vi "Conversion Lookup Table.vi"(6 "command":enum16{"Set All", "Lookup Parameters"}(ring), 8 "error in (no error)":errorcluster {"code" min=0 max=0}, 9 "ID":u32, 10 "J1939 Process Parameters":T3={"J1939 XNET Settings"={"XNET Database"="", "XNET Cluster"="", "CAN Port"="", "Baud rate [Bd]"=0, "Termination"=0, "Incoming Rate"=0, "Outcoming Rate"=1, "Write Decimation"=1}, "Incoming Single Point Configuraiton"={"Incoming Single Point Frame"={"ID"=[], "Conversion"=[], "Channel Array Positions"=[], "Frame Length"=[]}, "Channel Pairs"={"Chan Refs"=[], "Previous Chan Values"=[]}, "Read FIFO"=refnum}, "Outgoing Cyclic Configuraiton"={"Outgoing Cyclic Frame"={"ID"=[], "Conversion"=[], "Channel Array Positions"=[], "Frame Length"=[], "Transmit Propreties"=[]}, "Channel Pairs"={"Block Data Refs"=[], "Previous Chan Values"=[]}, "Write FIFO"=refnum}, "J1939 Monitor Settings"={"J1939 Network Address"=0, "Name"=0}, "Simulated Addresses"=[], "Simulated Addresses LUT"=variant, "Name"=""} {"Simulated Addresses"."Simulated Addresses"."J1939 XNET Settings"."Name" format="%.0x"; "Simulated Addresses"."Simulated Addresses"."DM1 Data"."Data Reference" format="%.0x"; "Simulated Addresses"."Simulated Addresses"."DM1 Enable?"."Data Reference" format="%.0x"; "Simulated Addresses"."Simulated Addresses"."DM2 Data"."Data Reference" format="%.0x"; "Simulated Addresses"."Simulated Addresses"."DM2 Enable?"."Data Reference" format="%.0x"; "J1939 Monitor Settings"."Name" format="%.0x"; "Outgoing Cyclic Configuraiton"."Channel Pairs"."Block Data Refs"."Data Reference" format="%.0x"; "Outgoing Cyclic Configuraiton"."Outgoing Cyclic Frame"."Transmit Propreties"."Transmit Time" format="%#_p"; "J1939 XNET Settings"."Termination" items=["Off", "On"]; "Incoming Single Point Configuraiton"."Channel Pairs"."Chan Refs" format="%.0x"}, 11 "Scale Ref":T1) -> (0 "error out":errorcluster {"code" min=0 max=0}, 1 "Found?":bool, 2 "Parameters":T2, 3 "Scale Ref out":T1)   [LabVIEW 2015, in "J1939 Addon Engine.lvlib"]
uses:
  J1939 Addon Engine.lvlib
  Types/Process Parameters.ctl
  Shared/Types/XNET Settings.ctl
  Types/Incoming Single Point Configuration.ctl
  Types/Incoming Single Point Frame Pairs.ctl
  Shared/Types/Incoming Single Point Channel Pairs.ctl
  <vilib>/NI Veristand/Custom Device API/Data Reference.ctl
  Types/Outgoing Cyclic Configuration.ctl
  Types/Outgoing Cyclic Frame Pairs.ctl
  Shared/Types/XNET Frame Event Properties.ctl
  Shared/Types/Outgoing Cyclic Channel Pairs.ctl
  <vilib>/NI Veristand/Custom Device API/Block Data Reference.ctl
  Shared/Types/Monitor Settings.ctl
  Types/Simulated Settings.ctl
  Shared/Types/Compiled Simulated Settings.ctl
  Types/DTC FIFOs.ctl
  Types/Conversion Lookup Table Parameters Cluster.ctl
  Types/Conversion Lookup Table Reference.ctl
  Shared/J1939 Utilities/SubVIs/Convert CAN Arb ID to J1939 ID.vi
  Shared/J1939 Utilities/J1939 Utilities.lvlib
  <vilib>/NI VeriStand/Custom Device API/Custom Device API.lvlib
  Shared/J1939 Addon Shared.lvlib
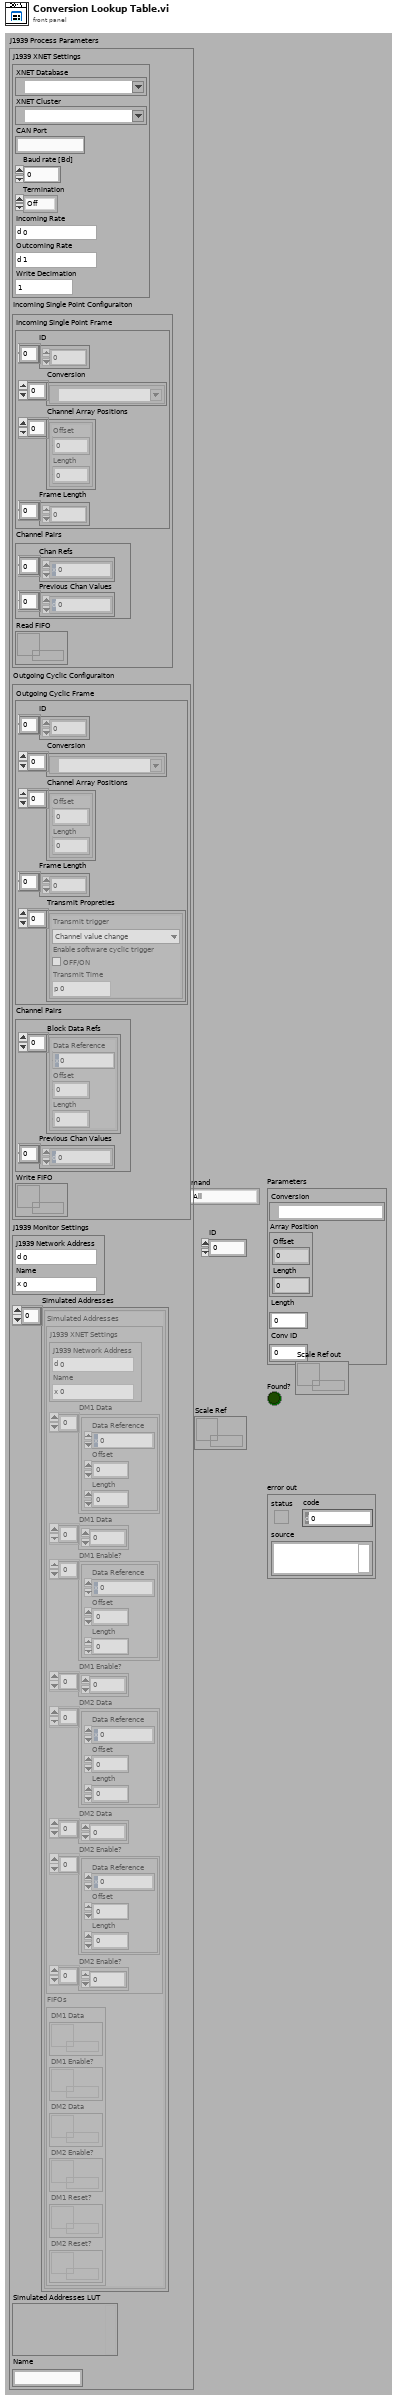
[diagram p1: front panel]
types:
  T1 = typedef "J1939 Addon Engine.lvlib/Conversion Lookup Table Reference.ctl" = refnum<data-value>
  T2 = typedef "J1939 Addon Engine.lvlib/Conversion Lookup Table Parameters Cluster.ctl" = cluster{"Conversion":refnum<k21>, "Array Position":cluster{"Offset":u32, "Length":u32}, "Length":u32, "Conv ID":u32}
  T3 = typedef "J1939 Addon Engine.lvlib/Process Parameters.ctl" = cluster{"J1939 XNET Settings":T4, "Incoming Single Point Configuraiton":T5, "Outgoing Cyclic Configuraiton":T9, "J1939 Monitor Settings":T14, "Simulated Addresses":T15[], "Simulated Addresses LUT":variant, "Name":string}
  T4 = typedef "J1939 Addon Shared.lvlib/XNET Settings.ctl" = cluster{"XNET Database":refnum<k21>, "XNET Cluster":refnum<k21>, "CAN Port":string, "Baud rate [Bd]":u32, "Termination":u32, "Incoming Rate":u32, "Outcoming Rate":u32, "Write Decimation":u32}
  T5 = typedef "J1939 Addon Engine.lvlib/Incoming Single Point Configuration.ctl" = cluster{"Incoming Single Point Frame":T6, "Channel Pairs":T7, "Read FIFO":refnum<k33>}
  T6 = typedef "J1939 Addon Engine.lvlib/Incoming Single Point Frame Pairs.ctl" = cluster{"ID":u32[], "Conversion":refnum<k21>[], "Channel Array Positions":cluster{"Offset":u32, "Length":u32}[], "Frame Length":u32[]}
  T7 = typedef "J1939 Addon Shared.lvlib/Incoming Single Point Channel Pairs.ctl" = cluster{"Chan Refs":T8[], "Previous Chan Values":dbl[]}
  T8 = typedef "Custom Device API.lvlib/Data Reference.ctl" = i32
  T9 = typedef "J1939 Addon Engine.lvlib/Outgoing Cyclic Configuration.ctl" = cluster{"Outgoing Cyclic Frame":T10, "Channel Pairs":T12, "Write FIFO":refnum<k33>}
  T10 = typedef "J1939 Addon Engine.lvlib/Outgoing Cyclic Frame Pairs.ctl" = cluster{"ID":u32[], "Conversion":refnum<k21>[], "Channel Array Positions":cluster{"Offset":u32, "Length":u32}[], "Frame Length":u32[], "Transmit Propreties":T11[]}
  T11 = typedef "J1939 Addon Shared.lvlib/XNET Frame Event Properties.ctl" = cluster{"Transmit trigger":enum16{"Channel value change"}, "Enable software cyclic trigger":bool, "Transmit Time":dbl}
  T12 = typedef "J1939 Addon Shared.lvlib/Outgoing Cyclic Channel Pairs.ctl" = cluster{"Block Data Refs":T13[], "Previous Chan Values":dbl[]}
  T13 = typedef "Custom Device API.lvlib/Block Data Reference.ctl" = cluster{"Data Reference":T8, "Offset":u64, "Length":u64}
  T14 = typedef "J1939 Addon Shared.lvlib/Monitor Settings.ctl" = cluster{"J1939 Network Address":u8, "Name":u64}
  T15 = typedef "J1939 Addon Engine.lvlib/Simulated Settings.ctl" = cluster{"Simulated Addresses":T16, "FIFOs":T17}
  T16 = typedef "J1939 Addon Shared.lvlib/Compiled Simulated Settings.ctl" = cluster{"J1939 XNET Settings":T14, "DM1 Data":T13[], "DM1 Data":dbl[], "DM1 Enable?":T13[], "DM1 Enable?":dbl[], "DM2 Data":T13[], "DM2 Data":dbl[], "DM2 Enable?":T13[], "DM2 Enable?":dbl[]}
  T17 = typedef "J1939 Addon Engine.lvlib/DTC FIFOs.ctl" = cluster{"DM1 Data":refnum<k33>, "DM1 Enable?":refnum<k33>, "DM2 Data":refnum<k33>, "DM2 Enable?":refnum<k33>, "DM1 Reset?":refnum<k33>, "DM2 Reset?":refnum<k33>}
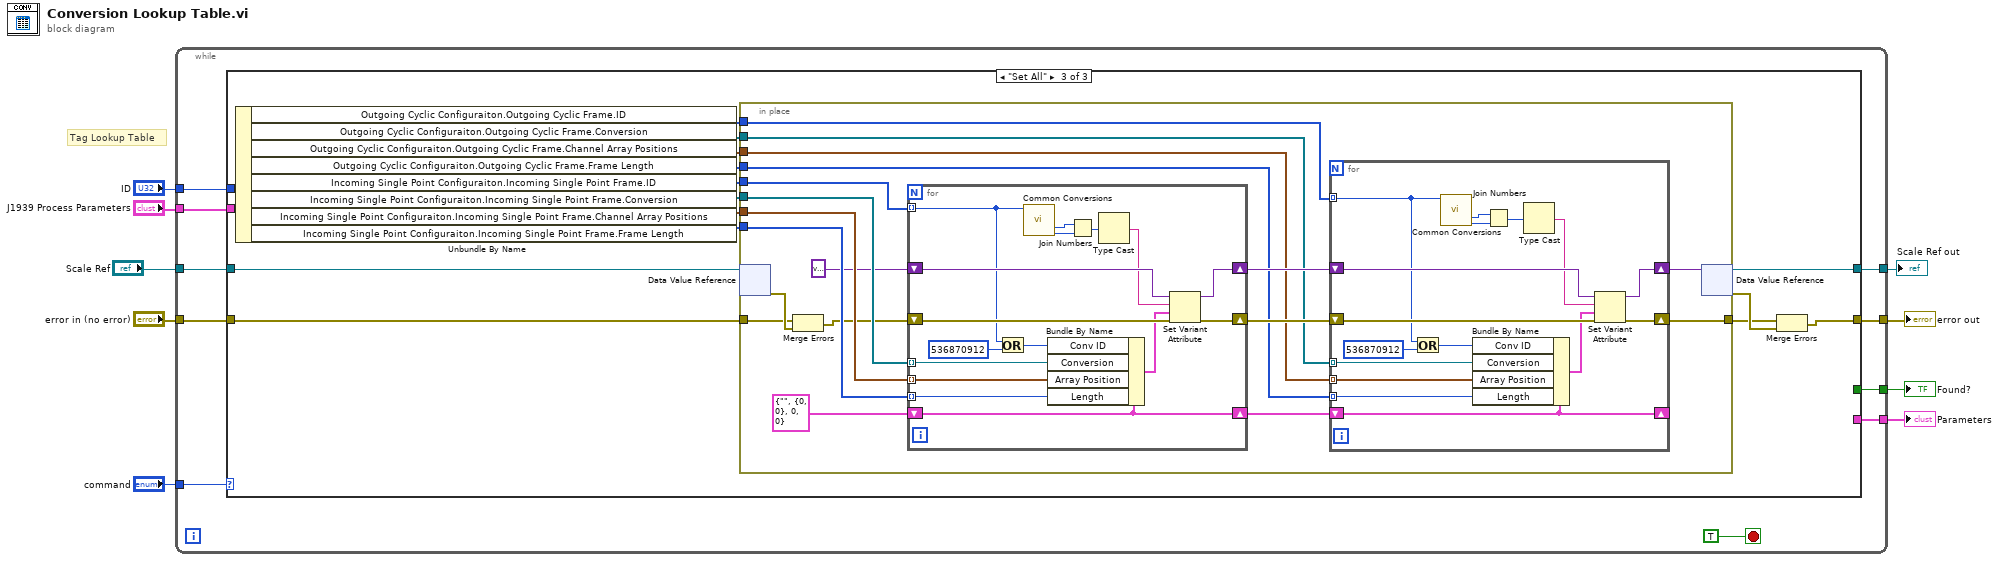
[diagram p0: block diagram]
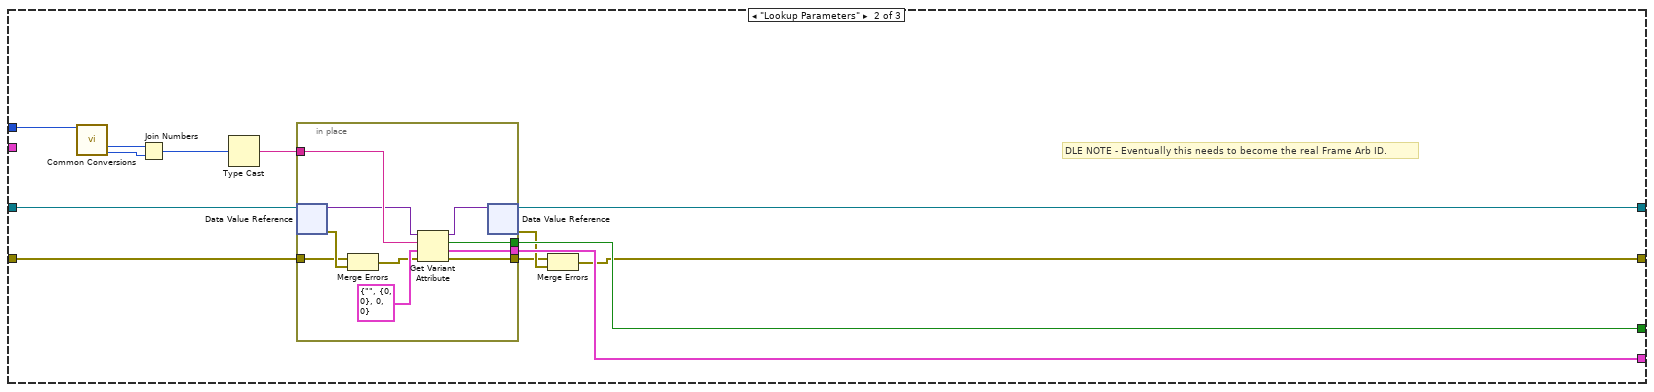
[diagram p3: hidden frame]
diagram:
  # "Tag Lookup Table"
  n1 = while {
    tunnel: "command" -> [w18]
    tunnel: "error in (no error)" -> [w17]
    tunnel: [w16] -> w7
    tunnel: "J1939 Process Parameters" -> [w15]
    tunnel: "ID" -> [w14]
    tunnel: [w13] -> w4
    tunnel: [w12] -> w3
    tunnel: "Scale Ref" -> [w11]
    tunnel: [w10] -> w1
    stop <- TRUE stop-if-true
    n2 = case shown="\"Set All\"" w18 {
      tunnel: w17 -> [w21 w34 w59]
      tunnel: [w21 w24 w47] -> w16
      tunnel: w15 -> [_ _ w58]
      tunnel: w14 -> [_ w31 _]
      tunnel: [_ w32 _] -> w13
      tunnel: [_ w29 _] -> w12
      tunnel: w11 -> [w20 w26 w49]
      tunnel: [w20 w22 w45] -> w10
      frame Default {
      }
      frame "Lookup Parameters" {
        # "DLE NOTE - Eventually this needs to become the real Frame Arb ID."
        n3 = call-poly "Common Conversions.vi"("Arb ID"=w31) -> ("PGN"=w30:u32, "Source Address"=w27:u8)  [unwired: 13 out]
        n4 = Join Numbers(hi=w30, lo=w27) -> ((hi.lo)=w28:u64)
        n5 = Type Cast(x=w28) -> (*(type *) &x=w33:string)  [unwired: 1 in]
        n6 = in-place {
          in-place-border: w34 -> [w36]
          in-place-border: w33 -> [w44]
          in-place-border: [w43] -> w23
          in-place-border: [w42] -> w32
          in-place-border: [w40] -> w29
          n7 = in-place-dvr #1(w26) -> (w39:variant, w37:errorcluster)
          n8 = Merge Errors(w36, w37) -> (w35:errorcluster)
          n9 = Get Variant Attribute(Variant=w39, name=w44, default value (empty Variant)=T2 {"Conversion"="", "Array Position"={"Offset"=0, "Length"=0}, "Length"=0, "Conv ID"=0} ("Parameters"), error in=w35) -> (duplicate Variant=w38:variant, found=w40:bool, value=w42:T2, error out=w43:errorcluster)
          n10 = in-place-dvr #1(w38) -> (w22:T1, w25:errorcluster)
        }
        n11 = Merge Errors(w23, w25) -> (w24:errorcluster)
      }
      frame "Set All" {
        n12 = Unbundle By Name(w58) -> ("Outgoing Cyclic Configuraiton.Outgoing Cyclic Frame.ID"=w53:u32[], "Outgoing Cyclic Configuraiton.Outgoing Cyclic Frame.Conversion"=w52:refnum<k21>[], "Outgoing Cyclic Configuraiton.Outgoing Cyclic Frame.Channel Array Positions"=w50:cluster{"Offset":u32, "Length":u32}[], "Outgoing Cyclic Configuraiton.Outgoing Cyclic Frame.Frame Length"=w51:u32[], "Incoming Single Point Configuraiton.Incoming Single Point Frame.ID"=w57:u32[], "Incoming Single Point Configuraiton.Incoming Single Point Frame.Conversion"=w56:refnum<k21>[], "Incoming Single Point Configuraiton.Incoming Single Point Frame.Channel Array Positions"=w55:cluster{"Offset":u32, "Length":u32}[], "Incoming Single Point Configuraiton.Incoming Single Point Frame.Frame Length"=w54:u32[])
        n13 = in-place {
          in-place-border: w59 -> [w61]
          in-place-border: w57 -> [w77]
          in-place-border: w56 -> [w76]
          in-place-border: w55 -> [w74]
          in-place-border: w54 -> [w73]
          in-place-border: [w70] -> w46
          in-place-border: w53 -> [w68]
          in-place-border: w52 -> [w67]
          in-place-border: w51 -> [w66]
          in-place-border: w50 -> [w65]
          n14 = in-place-dvr #2(w49) -> (w62:errorcluster)  [unwired: 1 out]
          n15 = Merge Errors(w61, w62) -> (w60:errorcluster)
          n16 = for {
            shift-right: [w108] -> w72
            shift-left: variant ("variant") -> [w109]
            shift-right: [w106] -> w71
            shift-left: w60 -> [w107]
            tunnel: w77 -> [w98] mode=indexing
            tunnel: w76 -> [w104] mode=indexing
            tunnel: w74 -> [w102] mode=indexing
            tunnel: w73 -> [w101] mode=indexing
            shift-right: [w100] -> w69
            shift-left: T2 {"Conversion"="", "Array Position"={"Offset"=0, "Length"=0}, "Length"=0, "Conv ID"=0} ("Parameters") -> [w100]
            n17 = Or(x=w98, y=u32 536870912) -> (x .or. y?=w97:u32)
            n18 = call-poly "Common Conversions.vi"("Arb ID"=w98) -> ("PGN"=w99:u32, "Source Address"=w94:u8)  [unwired: 13 out]
            n19 = Bundle By Name(cluster=w100, "Conv ID"=w97, "Conversion"=w104, "Array Position"=w102, "Length"=w101) -> (w103:T2)
            n20 = Join Numbers(hi=w99, lo=w94) -> ((hi.lo)=w95:u64)
            n21 = Type Cast(x=w95) -> (*(type *) &x=w105:string)  [unwired: 1 in]
            n22 = Set Variant Attribute(Variant=w109, name=w105, value=w103, error in=w107) -> (Variant out=w108:variant, error out=w106:errorcluster)  [unwired: 1 out]
          }
          n23 = for {
            shift-right: [w92] -> w63
            shift-left: w72 -> [w93]
            shift-right: [w90] -> w70
            shift-left: w71 -> [w91]
            tunnel: w68 -> [w82] mode=indexing
            tunnel: w67 -> [w88] mode=indexing
            tunnel: w65 -> [w86] mode=indexing
            tunnel: w66 -> [w85] mode=indexing
            shift-right: [w84] -> _
            shift-left: w69 -> [w84]
            n24 = Or(x=w82, y=u32 536870912) -> (x .or. y?=w81:u32)
            n25 = call-poly "Common Conversions.vi"("Arb ID"=w82) -> ("PGN"=w80:u32, "Source Address"=w79:u8)  [unwired: 13 out]
            n26 = Bundle By Name(cluster=w84, "Conv ID"=w81, "Conversion"=w88, "Array Position"=w86, "Length"=w85) -> (w87:T2)
            n27 = Join Numbers(hi=w80, lo=w79) -> ((hi.lo)=w78:u64)
            n28 = Type Cast(x=w78) -> (*(type *) &x=w89:string)  [unwired: 1 in]
            n29 = Set Variant Attribute(Variant=w93, name=w89, value=w87, error in=w91) -> (Variant out=w92:variant, error out=w90:errorcluster)  [unwired: 1 out]
          }
          n30 = in-place-dvr #2(w63) -> (w45:T1, w48:errorcluster)
        }
        n31 = Merge Errors(w46, w48) -> (w47:errorcluster)
      }
    }
  }
  "error out" <- w7
  "Parameters" <- w4
  "Found?" <- w3
  "Scale Ref out" <- w1
